vi "Is Remote Terminal.vi"(7 "RT1?":bool, 8 "error in (no error)":errorcluster, 11 "1553 SubComponent":refnum<class "1553 SubComponent.lvclass">) -> (0 "error out":errorcluster)   [LabVIEW 2020, in "BCI-1553 API.lvlib" / "1553 Component.lvclass"]
doc: "Checks if the component is configured as a remote terminal. Will report an error if the subcomponent is not a remote terminal."
uses:
  1553 Component.lvclass
  1553 SubComponent/1553 SubComponent.lvclass
  Remote Terminal/Remote Terminal.lvclass
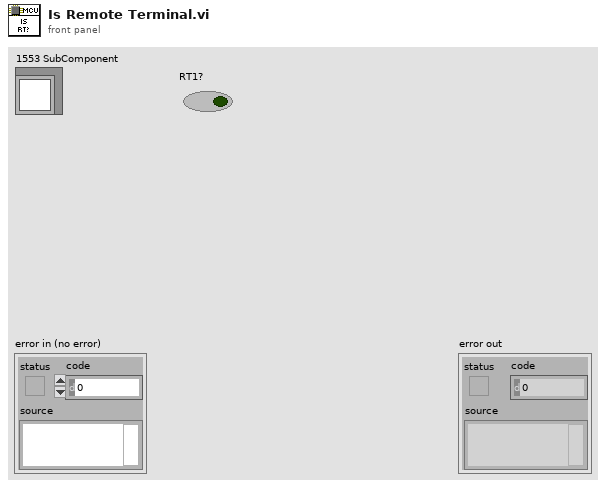
[diagram p1: front panel]
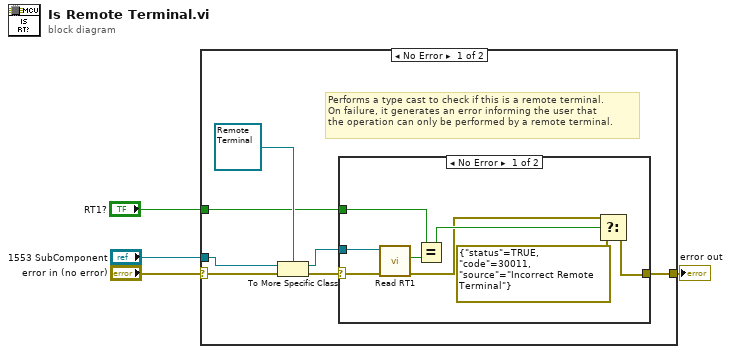
[diagram p0: block diagram]
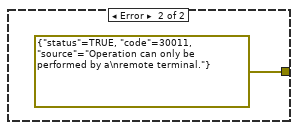
[diagram p2: hidden frame]
diagram:
  n1 = case shown="No Error" "error in (no error)" {
    selector: "error in (no error)" -> [w9 w21]
    tunnel: [w11 w21] -> w3
    tunnel: "1553 SubComponent" -> [w10 _]
    tunnel: "RT1?" -> [w6 _]
    frame No Error {
      # "Performs a type cast to check if this is a remote terminal.\nOn failure, it generates an error informing the user that\nthe operation can only be performed by a remote terminal."
      n2 = To More Specific Class(target class=refnum<class "Remote Terminal.lvclass"> refnum ("SLSC 1553 API.lvlib:Remote Terminal.lvclass"), reference=w10, error in=w9) -> (specific class reference=w5:refnum<class "Remote Terminal.lvclass">, error out=w8:errorcluster)
      n3 = case shown="No Error" w8 {
        selector: w8 -> [w18 _]
        tunnel: [w13 errorcluster {"status"=TRUE, "code"=30011, "source"="Operation can only be performed by a\nremote terminal."} ("error IO")] -> w11
        tunnel: w6 -> [w16 _]
        tunnel: w5 -> [w19 _]
        frame No Error {
          n4 = call-dynamic "Read RT1.vi"("error in (no error)"=w18, "Remote Terminal in"=w19) -> ("error out"=w14:errorcluster, "RT1"=w17:bool)  [unwired: 7 in, 1 out]
          n5 = Equal?(x=w16, y=w17) -> (x = y?=w15:bool)
          n6 = Select(t=w14, s=w15, f=errorcluster {"status"=TRUE, "code"=30011, "source"="Incorrect Remote Terminal"}) -> (s? t:f=w13:errorcluster)
        }
        frame Error {
        }
      }
    }
    frame Error {
    }
  }
  "error out" <- w3
